vi "Node Change Event.vi"(8 "error in (no error)":errorcluster, 9 "Send (T)":bool=TRUE, 10 "objects":T8, 11 "References in":T1) -> (0 "error out":errorcluster)   [LabVIEW 2014, in "Calculated Tags editor node.lvclass"]
doc: "Notifies the background table manager service that a change to the table has occured."
uses:
  Calculated Tags editor node.lvclass
  <vilib>/NI/DCAF/Tag Editor Core/Table API/Table Manager/object ref.ctl
  <vilib>/NI/DCAF/Tag Editor Core/Configuration Editor/Classes/Engine Parent/Engine Parent Editor Node.lvclass
  <vilib>/NI/DCAF/Tag Editor Core/Configuration Editor/Classes/Module editor node/module editor node.lvclass
  <vilib>/NI/DCAF/Tag Editor Core/Table API/Table Manager/references.ctl
  <vilib>/NI/Configuration Framework/Node/StopEvent.ctl
  <vilib>/NI/Configuration Framework/Node/RefreshUIEvent.ctl
  <vilib>/NI/Configuration Framework/Node/CacheState.ctl
  <vilib>/NI/Configuration Framework/Node/NodeChangeEvent.ctl
  <vilib>/NI/Configuration Framework/Node/NodeRef.ctl
  <vilib>/NI/Configuration Framework/Node/NISE_CEF_Node.lvclass
  <vilib>/NI/DCAF/Tag Editor Core/Table API/Available Tag Menu/channel action event.ctl
  <vilib>/NI/DCAF/Tag Editor Core/Table API/Available Tag Menu/dialog output action.ctl
  <vilib>/NI/Tag Bus Module Framework/channel/TBM channel.lvclass
  <vilib>/NI/Tag Bus/tag/tag descriptor.lvclass
  <vilib>/NI/DCAF/Tag Editor Core/Table API/Table Manager/Call Back Ref Type Def.ctl
  <vilib>/NI/AMC/Message Queue.ctl
  <vilib>/NI/AMC/Message.ctl
  <vilib>/NI/Tools/Keyed Array/KeyedArray.ctl
  <vilib>/NI/Configuration Framework/Node/UserEventRef.ctl
  <vilib>/NI/Configuration Framework/Controls/EventCluster.ctl
  <vilib>/NI/DCAF/Tag Editor Core/Table API/Table Manager/Table Manager.lvclass
  <vilib>/NI/DCAF/Tag Editor Core/Table API/Table Manager.lvlib
  <vilib>/NI/Tools/Keyed Array/Tools_KeyedArray.lvlib
  <vilib>/NI/AMC/AMC.lvlib
  <vilib>/NI/Configuration Framework/NISE_CEF_TreeControl.lvlib
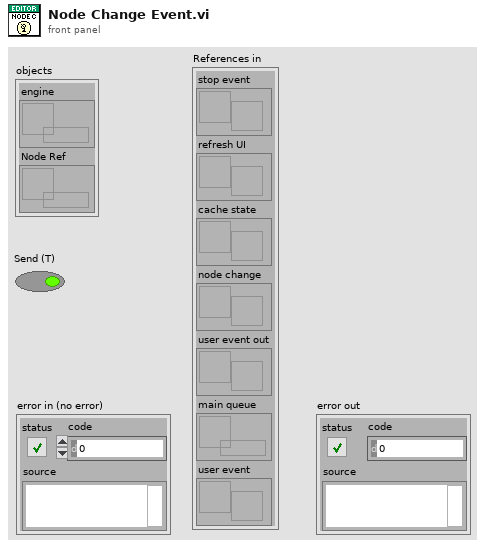
[diagram p1: front panel]
types:
  T1 = typedef "Table Manager.lvlib/Table Manager.lvclass/references.ctl" = cluster{"stop event":T2, "refresh UI":T3, "cache state":T4, "node change":T5, "user event out":refnum<user-event>, "main queue":T6, "user event":T7}
  T2 = typedef "NISE_CEF_Node.lvclass/StopEvent.ctl" = refnum<user-event>
  T3 = typedef "NISE_CEF_Node.lvclass/RefreshUIEvent.ctl" = refnum<user-event>
  T4 = typedef "NISE_CEF_Node.lvclass/CacheState.ctl" = refnum<user-event>
  T5 = typedef "NISE_CEF_Node.lvclass/NodeChangeEvent.ctl" = refnum<user-event>
  T6 = typedef "AMC.lvlib/Message Queue.ctl" = refnum<queue>
  T7 = typedef "NISE_CEF_Node.lvclass/UserEventRef.ctl" = refnum<user-event>
  T8 = typedef "Table Manager.lvlib/Table Manager.lvclass/object ref.ctl" = cluster{"engine":refnum<data-value>, "Node Ref":refnum<data-value>}
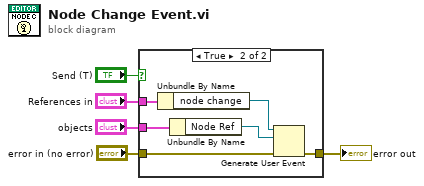
[diagram p0: block diagram]
diagram:
  n1 = case shown="True" "Send (T)" {
    tunnel: "References in" -> [_ w12]
    tunnel: "objects" -> [_ w10]
    tunnel: "error in (no error)" -> [w6 w8]
    tunnel: [w6 w7] -> w2
    frame False {
    }
    frame True {
      n2 = Unbundle By Name(w12) -> ("node change"=w11:T5)
      n3 = Unbundle By Name(w10) -> ("Node Ref"=w9:refnum<data-value>)
      n4 = Generate User Event(user event=w11, event data cluster=w9, error in=w8) -> (error out=w7:errorcluster)  [unwired: 1 in, 1 out]
    }
  }
  "error out" <- w2
